vi "OpenMVTestCode.vi"() -> ()   [LabVIEW 2016]
panel:
  out "new picture":picture
  out "Array 4":bool[](array[boolean])
  out "Time":u32[](array[numeric])
  out "length read":i32[](array[numeric])
  out "size()":u32[][](array[numeric])
  out "Excess bytes":i32[](array[numeric])
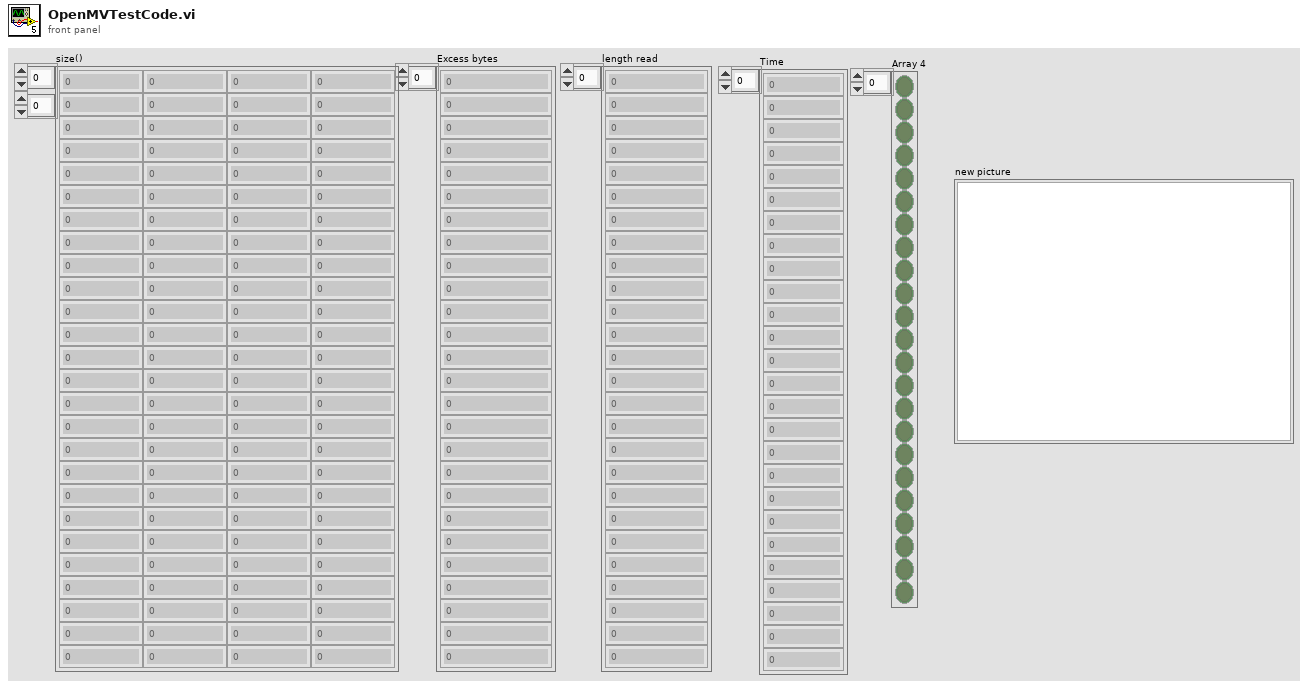
[diagram p1: front panel]
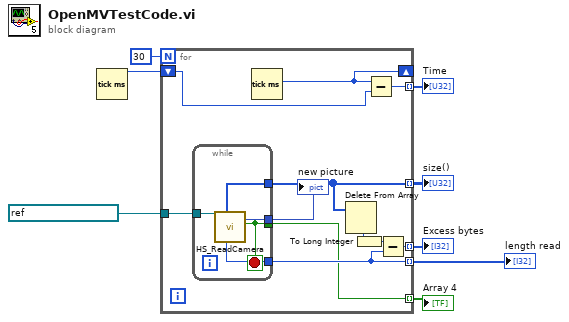
[diagram p0: block diagram]
diagram:
  n1 = Tick Count (ms)() -> (millisecond timer value=w2:u32)
  n2 = for {
    N: 30 -> [_]
    tunnel: [w19] -> w6 mode=indexing
    tunnel: [w17] -> w5 mode=indexing
    tunnel: [w16] -> w7 mode=indexing
    tunnel: refnum<visa-resource-name> "ASRL12::INSTR" ("VISA Refnum in") -> [w15]
    tunnel: [w13] -> w3 mode=indexing
    shift-right: [w12] -> _
    shift-left: w2 -> [w11]
    tunnel: [w10] -> w1 mode=indexing
    n3 = while {
      tunnel: [w24] -> w19
      tunnel: [w23] -> w17
      tunnel: w15 -> [w22]
      tunnel: [w20] -> w10
      tunnel: [w21] -> w9
      stop <- w20 stop-if-true
      n4 = call "HS_ReadCamera.vi"("VISA Refnum in"=w22) -> ("Good?"=w20:bool, "new picture"=w21:picture, "length"=w23:i32, "size()"=w24:u32[])  [unwired: 3 in, 4 out]
    }
    "new picture" <- w9
    n5 = Tick Count (ms)() -> (millisecond timer value=w12:u32)
    n6 = Delete From Array(array=w19) -> (deleted portion=w18:u32)  [unwired: 2 in, 1 out]
    n7 = To Long Integer(number=w18) -> (32bit integer=w14:i32)
    n8 = Subtract(x=w12, y=w11) -> (x-y=w13:u32)
    n9 = Subtract(x=w14, y=w17) -> (x-y=w16:i32)
  }
  "Excess bytes" <- w7
  "size()" <- w6
  "length read" <- w5
  "Time" <- w3
  "Array 4" <- w1
